vi "Select PID Values.vi"(9 "Enum":enum16{"30V", "40V"}(ring)=enum."40V", 10 "current field":dbl[unit]) -> (2 "PID output":cluster{"I":dbl, "D":dbl, "P":dbl})   [LabVIEW 2009, in "Varian Magnet.lvclass"]
doc: "this returns the appropriate PID settings when the control voltage is 40V...change later to adapt to 30V settings too."
uses:
  Varian Magnet.lvclass
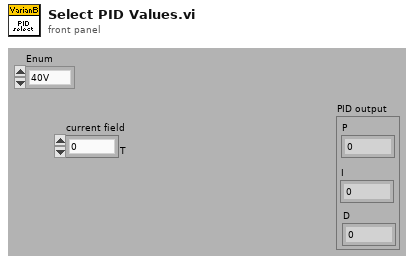
[diagram p1: front panel]
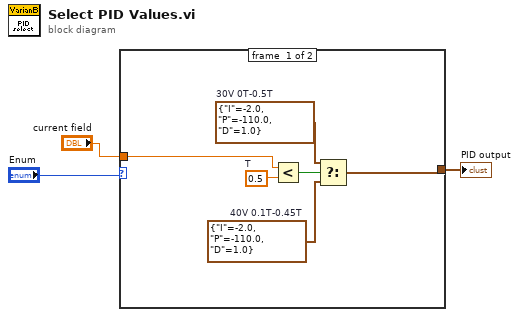
[diagram p0: block diagram]
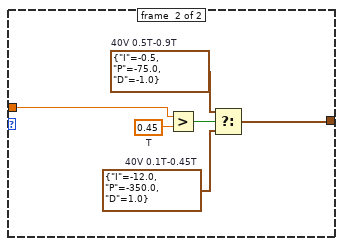
[diagram p2: hidden frame]
diagram:
  n1 = case shown="\"30V\"" "Enum" {
    tunnel: [w4 w11] -> w2
    tunnel: "current field" -> [w5 w10]
    frame #0 {
      w6 = cluster{"I":dbl, "P":dbl, "D":dbl} {"I"=-2.0, "P"=-110.0, "D"=1.0}  # 40V 0.1T-0.45T
      w7 = cluster{"I":dbl, "P":dbl, "D":dbl} {"I"=-2.0, "P"=-110.0, "D"=1.0}  # 30V 0T-0.5T
      w9 = dbl[unit] 0.5  # T
      n2 = Less?(x=w5, y=w9) -> (x < y?=w8:bool)
      n3 = Select(t=w7, s=w8, f=w6) -> (s? t:f=w4:cluster{"I":dbl, "P":dbl, "D":dbl})
    }
    frame #1 {
      w12 = cluster{"I":dbl, "P":dbl, "D":dbl} {"I"=-12.0, "P"=-350.0, "D"=1.0}  # 40V 0.1T-0.45T
      w13 = cluster{"I":dbl, "P":dbl, "D":dbl} {"I"=-0.5, "P"=-75.0, "D"=-1.0}  # 40V 0.5T-0.9T
      w15 = dbl[unit] 0.45  # T
      n4 = Greater?(x=w10, y=w15) -> (0:w14:bool)
      n5 = Select(t=w13, s=w14, f=w12) -> (s? t:f=w11:cluster{"I":dbl, "P":dbl, "D":dbl})
    }
  }
  "PID output" <- w2
